vi "DelArrayEndNumI32.vi"(8 "ErrorIn(No Error)":errorcluster caption="entrée d'erreur (pas d'erreur)", 10 "Array In":i32[](array[numeric]), 11 "Nombre":i32=-1) -> (0 "sortie d'erreur":errorcluster, 2 "Array Out":i32[](array[numeric]))   [LabVIEW 2012]
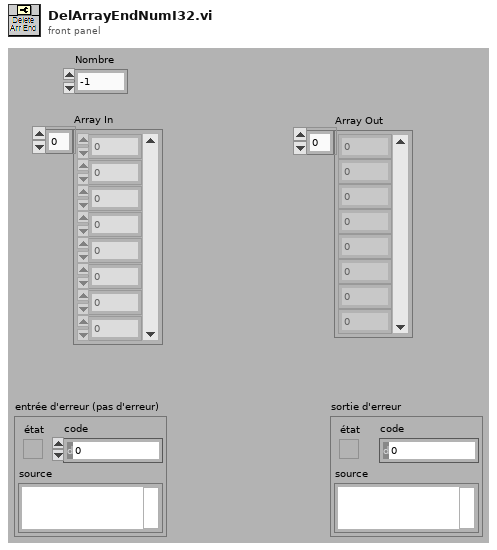
[diagram p1: front panel]
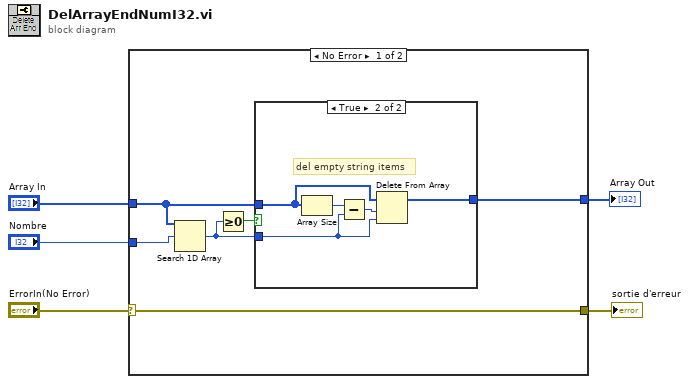
[diagram p0: block diagram]
diagram:
  n1 = case shown="No Error" "ErrorIn(No Error)" {
    selector: "ErrorIn(No Error)" -> [w11 w19]
    tunnel: [w11 w19] -> w4
    tunnel: "Array In" -> [w8 w18]
    tunnel: [w7 w18] -> w2
    tunnel: "Nombre" -> [w6 _]
    frame No Error {
      n2 = Search 1D Array(1D array=w8, element=w6) -> (index of element=w10:i32)  [unwired: 1 in]
      n3 = Greater Or Equal To 0?(x=w10) -> (x >= 0?=w9:bool)
      n4 = case shown="True" w9 {
        tunnel: w10 -> [_ w15]
        tunnel: w8 -> [w12 w13]
        tunnel: [w12 w14] -> w7
        frame False {
          # "no empty String found"
        }
        frame True {
          # "del empty string items"
          n5 = Array Size(array=w13) -> (size(s)=w17:i32)
          n6 = Subtract(x=w17, y=w15) -> (x-y=w16:i32)
          n7 = Delete From Array(array=w13, length=w16, index=w15) -> (array with subset deleted=w14:i32[])  [unwired: 1 out]
        }
      }
    }
    frame Error {
    }
  }
  "sortie d'erreur" <- w4
  "Array Out" <- w2
